vi "Read Session.vi"(8 "Error In":errorcluster, 11 "SFTP In":refnum<class "SFTP.lvclass">) -> (0 "Erorr Out":errorcluster, 2 "Session":refnum<class "Session.lvclass">, 3 "SFTP Out":refnum<class "SFTP.lvclass">)   [LabVIEW 2018, in "Toolkit.lvlib" / "SFTP.lvclass"]
doc: "Gets the Session used to create the SFTP object."
uses:
  SFTP.lvclass
  Session/Session.lvclass
  SFTP.lvclass/SFTP.ctl
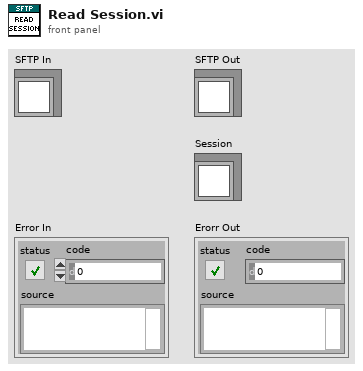
[diagram p1: front panel]
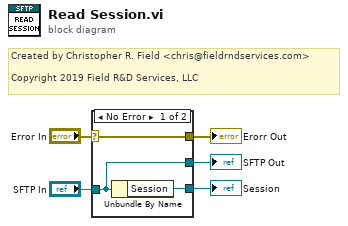
[diagram p0: block diagram]
diagram:
  # "Created by Christopher R. Field <chris@fieldrndservices.com>\n\nCopyright 2019 Field R&D Services, LLC"
  n1 = case shown="No Error" "Error In" {
    selector: "Error In" -> [w7 w9]
    tunnel: [w7 w9] -> w4
    tunnel: "SFTP In" -> [w8 w10]
    tunnel: [w8 w10] -> w2
    tunnel: [w6 _] -> w1
    frame No Error {
      n2 = Unbundle By Name(w8) -> ("Session"=w6:refnum<class "Session.lvclass">)
    }
    frame Error {
    }
  }
  "Erorr Out" <- w4
  "SFTP Out" <- w2
  "Session" <- w1
